vi "Get_Shaft_IT_Grade.vi"(8 "error in (no error)":errorcluster, 11 "Data Cluster in":T1 {"Shaft"."dmin" format="%#_7g"; "Shaft"."dmax" format="%#_7g"; "Shaft"."Fundamental Dev" format="%#_7g"; "Shaft"."Tolerance Grade (IT) Shaft" format="%#_7g"; "Hole"."Dmin" format="%#_7g"; "Hole"."Tolerance Grade (IT)" format="%#_7g"}) -> (0 "error out":errorcluster, 3 "Data Cluster out":T1 {"Shaft"."dmin" format="%#_7g"; "Shaft"."dmax" format="%#_7g"; "Shaft"."Fundamental Dev" format="%#_7g"; "Shaft"."Tolerance Grade (IT) Shaft" format="%#_7g"; "Hole"."Dmin" format="%#_7g"; "Hole"."Tolerance Grade (IT)" format="%#_7g"})   [LabVIEW 2023]
uses:
  TypeDef/Data_Cluster.ctl
  <vilib>/MGI/Panel Manager/Panel/Panel/Window/Window.lvclass
  TypeDef/Units.ctl
  TypeDef/Method_Info.ctl
  TypeDef/Hole_Data.ctl
  TypeDef/Shaft_Data.ctl
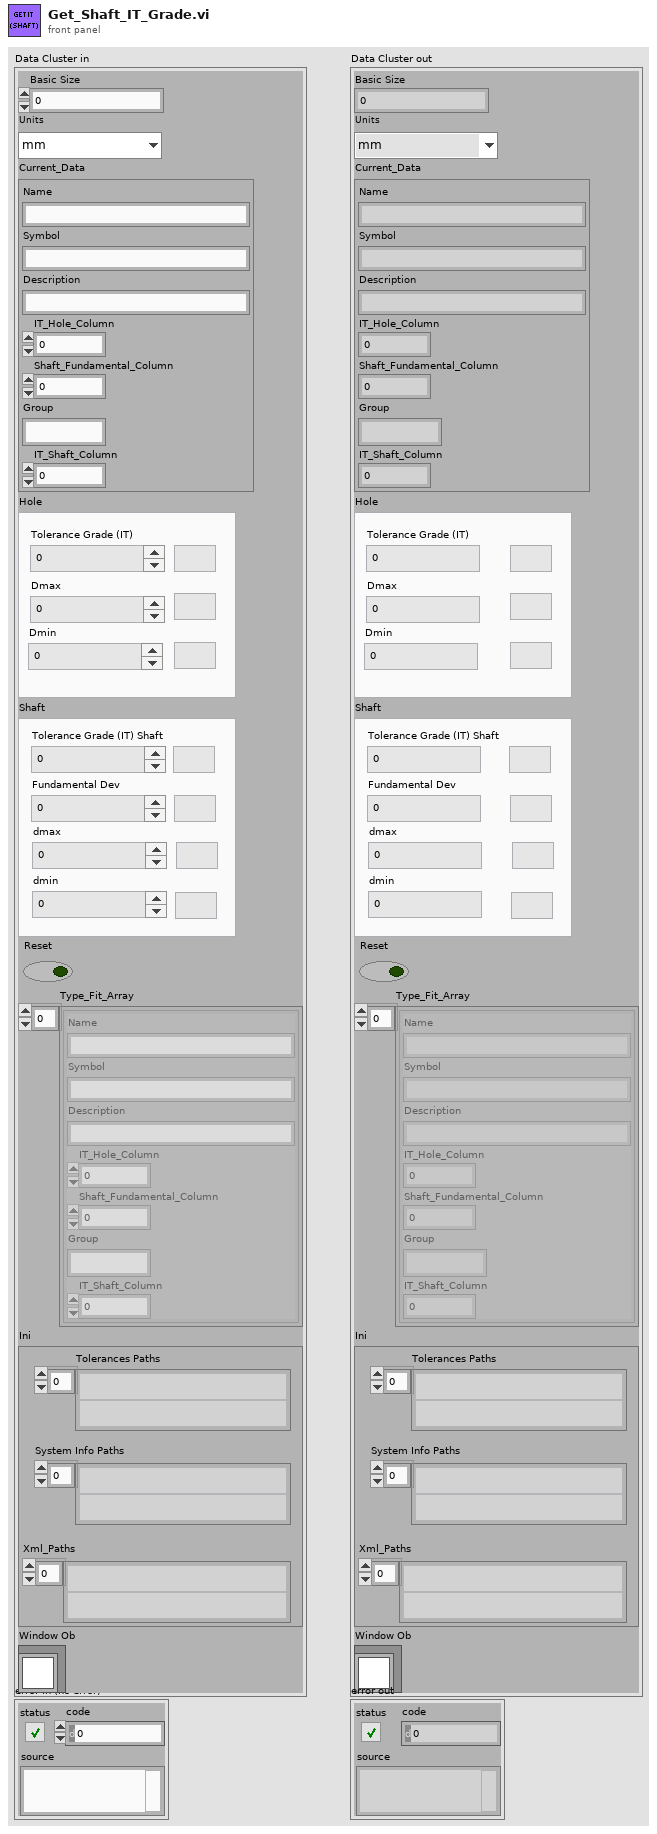
[diagram p1: front panel]
types:
  T1 = typedef "Data_Cluster.ctl" = cluster{"Basic Size ":dbl, "Units":T2, "Current_Data":T3, "Hole":T4, "Shaft":T5, "Reset":bool, "Type_Fit_Array":T3[], "Ini":cluster{"Tolerances Paths":path[], "System Info Paths":path[], "Xml_Paths":path[]}, "Window Ob":refnum<class "Window.lvclass">}
  T2 = typedef "Units.ctl" = enum16{"mm", "in"}
  T3 = typedef "Method_Info.ctl" = cluster{"Name":string, "Symbol":string, "Description":string, "IT_Hole_Column":i32, "Shaft_Fundamental_Column":i32, "Group":string, "IT_Shaft_Column":i32}
  T4 = typedef "Hole_Data.ctl" = cluster{"Tolerance Grade (IT)":dbl, "Dmax":dbl, "Units Hole":cluster{"units_it":string, "units_Dmax\nUnits_Dmax":string, "Units_Dmin":string}, "Dmin":dbl}
  T5 = typedef "Shaft_Data.ctl" = cluster{"Tolerance Grade (IT) Shaft":dbl, "Units Shaft":cluster{"Units_FundamentalDev":string, "Units_dmax":string, "Units_dmin":string, "Units_IT_Shaft":string}, "Fundamental Dev":dbl, "dmax":dbl, "dmin":dbl}
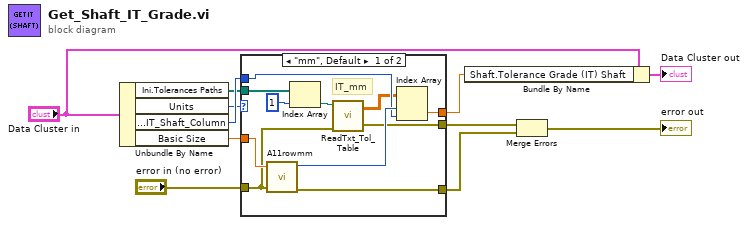
[diagram p0: block diagram]
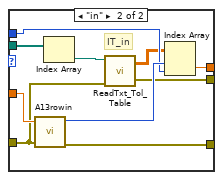
[diagram p2: hidden frame]
diagram:
  n1 = Unbundle By Name("Data Cluster in") -> ("Ini.Tolerances Paths"=w5:path[], "Units"=w2:T2, "Current_Data.IT_Shaft_Column"=w7:i32, "Basic Size"=w6:dbl)
  n2 = case shown="\"mm\", Default" w2 {
    tunnel: "error in (no error)" -> [w15 w26]
    tunnel: [w22 w32] -> w4
    tunnel: w5 -> [w14 w23]
    tunnel: w6 -> [w21 w31]
    tunnel: [w18 w30] -> w10
    tunnel: w7 -> [w19 w28]
    tunnel: [w16 w27] -> w9
    frame "mm", Default {
      # "IT_mm"
      n3 = call "A11rowmm.vi"("Basic Size"=w21, "error in (no error)"=w15) -> ("Row"=w20:i32, "error out"=w22:errorcluster)  [unwired: 5 in]
      n4 = Index Array(array=w14, index=1) -> (element=w13:path)
      n5 = call "ReadTxt_Tol_Table.vi"("error in"=w15, "ITmm path"=w13) -> ("error out"=w16:errorcluster, "array_of_tolerances"=w17:dbl[][])  [unwired: 4 in]
      n6 = Index Array(array=w17, index (row)=w20, index (col)=w19) -> (element=w18:dbl)
    }
    frame "in" {
      # "IT_in"
      n7 = call "A13rowin.vi"("Basic Size"=w31, "error in"=w26) -> ("Row"=w29:i32, "error out"=w32:errorcluster)  [unwired: 5 in]
      n8 = Index Array(array=w23) -> (element=w24:path)  [unwired: 1 in]
      n9 = call "ReadTxt_Tol_Table.vi"("error in"=w26, "ITmm path"=w24) -> ("error out"=w27:errorcluster, "array_of_tolerances"=w25:dbl[][])  [unwired: 4 in]
      n10 = Index Array(array=w25, index (row)=w29, index (col)=w28) -> (element=w30:dbl)
    }
  }
  n11 = Bundle By Name(cluster="Data Cluster in", "Shaft.Tolerance Grade (IT) Shaft"=w10) -> (→"Data Cluster out":T1)
  n12 = Merge Errors(w9, w4) -> (→"error out":errorcluster)
